vi "Update.vi"(4 "Value2":dbl, 6 "Value1":dbl, 8 "error in (no error)":errorcluster, 9 "Audio History Buffer In":dbl[][](array[numeric]), 10 "Audio Data In":dbl[][](array[numeric]), 11 "Effect Interface in":refnum<class "Effect Interface.lvclass">) -> (0 "error out":errorcluster, 1 "Audio History Buffer Out":dbl[][](array[numeric]), 2 "Audio Data Out":dbl[][](array[numeric]), 3 "Effect Interface out":refnum<class "Effect Interface.lvclass">)   [LabVIEW 2019, in "Effect Interface.lvlib" / "Effect Interface.lvclass"]
doc: "Run the effect processing.\n\nThis is an Interface VI. Effect plugins need to override this VI."
uses:
  Effect Interface.lvclass
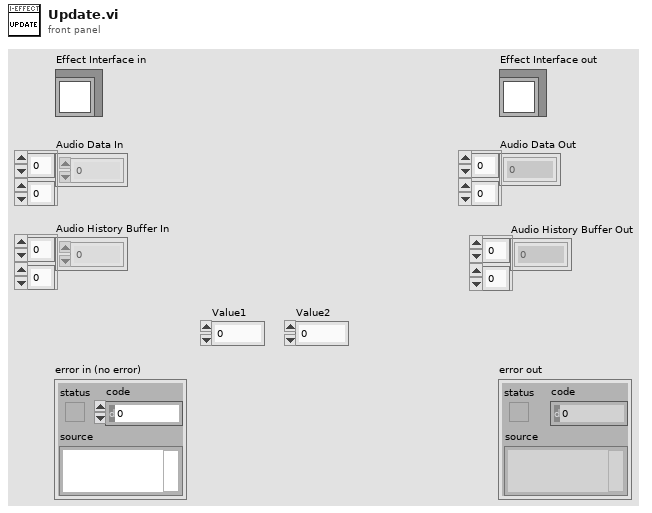
[diagram p1: front panel]
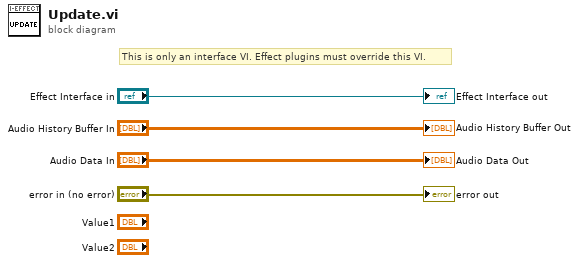
[diagram p0: block diagram]
diagram:
  # "This is only an interface VI. Effect plugins must override this VI."
  "Audio Data Out" <- "Audio Data In"
  "error out" <- "error in (no error)"
  "Effect Interface out" <- "Effect Interface in"
  "Audio History Buffer Out" <- "Audio History Buffer In"
